vi "speed encoder trial.vi"() -> ()   [LabVIEW 2018]
panel:
  in  "new value":dbl format="%#_13g"
  in  "average":dbl=75500.0 format="%#_13g"
  out "result":dbl
  out "XY Graph":T1(graph)
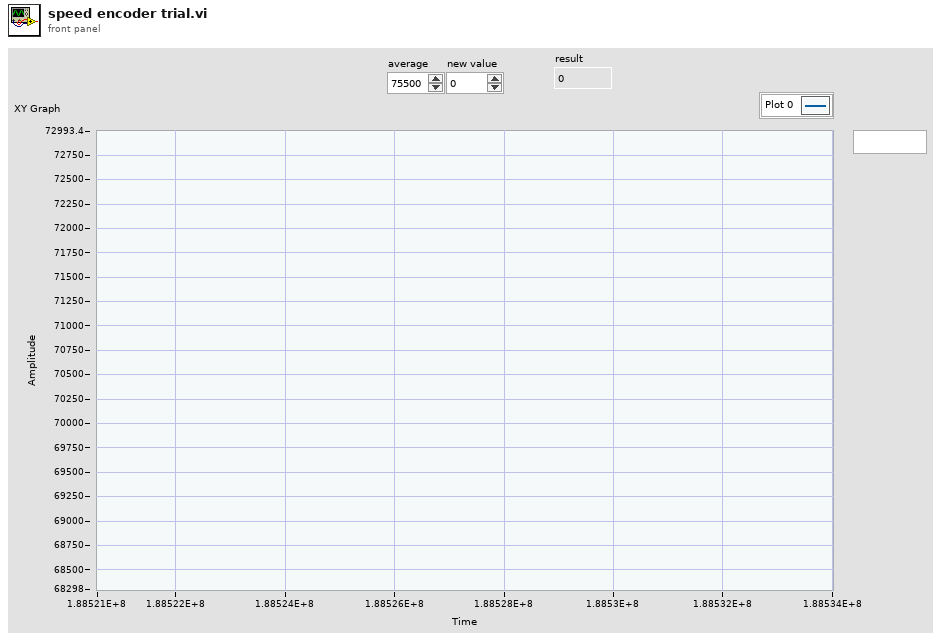
[diagram p1: front panel]
types:
  T1 = cluster{"Data received":sgl[], "Data received":sgl[]}[]
  T2 = cluster{"Data received":sgl[], "Data received":sgl[]}
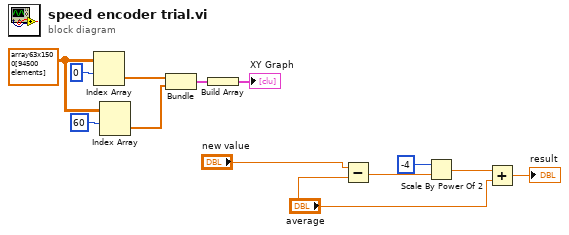
[diagram p0: block diagram]
diagram:
  w7 = sgl[][] array63x1500[94500 elements] ("Data received")
  n1 = Index Array(array=w7, index (row)=0) -> (element=w10:sgl[])  [unwired: 1 in]
  n2 = Index Array(array=w7, index (row)=60) -> (element=w11:sgl[])  [unwired: 1 in]
  n3 = Bundle("Data received"=w10, "Data received"=w11) -> (w9:T2)  [unwired: 1 in]
  n4 = Build Array(w9) -> (→"XY Graph":T1)
  n5 = Subtract(x="new value", y="average") -> (x-y=w5:dbl)
  n6 = Scale By Power Of 2(n=i16 -4, x=w5) -> (x*2^n=w3:dbl)
  n7 = Add(x=w3, y="average") -> (x+y=→"result":dbl)
